vi "config_string_to_toml_string.vi"(8 "error in (no error)":errorcluster, 11 "Config String (\"\") in":string) -> (0 "error out":errorcluster, 3 "toml":string)   [LabVIEW 2020]
uses:
  2655c186-cb49-4fe9-925e-dcd75411c460.vi
  configuration-data/configuration-data.lvclass
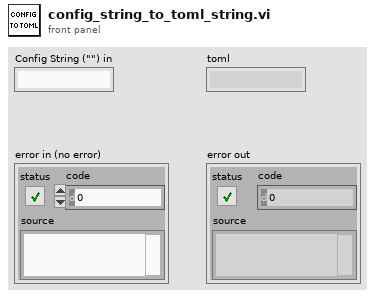
[diagram p1: front panel]
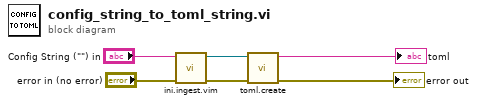
[diagram p0: block diagram]
diagram:
  n1 = call "ini.ingest.vim"("error in"="error in (no error)", "config string or path"="Config String (\"\") in") -> ("error out"=w4:errorcluster, "configuration-data"=w5:refnum<class "configuration-data.lvclass">)  [unwired: 8 in]
  n2 = call "toml.create.vi"("error in"=w4, "configuration-data"=w5) -> ("error out"=→"error out":errorcluster, "toml"=→"toml":string)  [unwired: 8 in]
